vi "read_db_for_batch_processor.vi"(7 "Update Error files?":bool, 8 "error in (no error)":errorcluster, 9 "Lower Timestamp":timestamp, 10 "Upper Timestamp":timestamp, 11 "Update old files?":bool) -> (0 "error out":errorcluster, 3 "BP Array":T1[](array[typedef]) {"File Location" items=["Currently Writing"=-3, "Labview Files"=-2, "Mars Data Processing Factility"=-1, "Local Cache "=0, "Old Storage"=1, "Storage"=2]})   [LabVIEW 2012]
uses:
  Batch Processor/bp_cluster.ctl
  File_location.ctl
  <vilib>/addons/database/Auxilliary.llb/DB Tools Cursor Type.ctl
  <vilib>/addons/database/Connection.llb/Conn Execute.vi
  <vilib>/addons/database/Recordset.llb/Rec Fetch Recordset Data (R).vi
  <vilib>/addons/database/Recordset.llb/Rec Destroy - Connection.vi
  <vilib>/addons/database/_DB Variant To Data/Database Variant To Data.xnode
  <vilib>/addons/database/NI_Database_API.lvlib
panel:
  out "size(s)":i32
  out "SQL Query Sintax":string
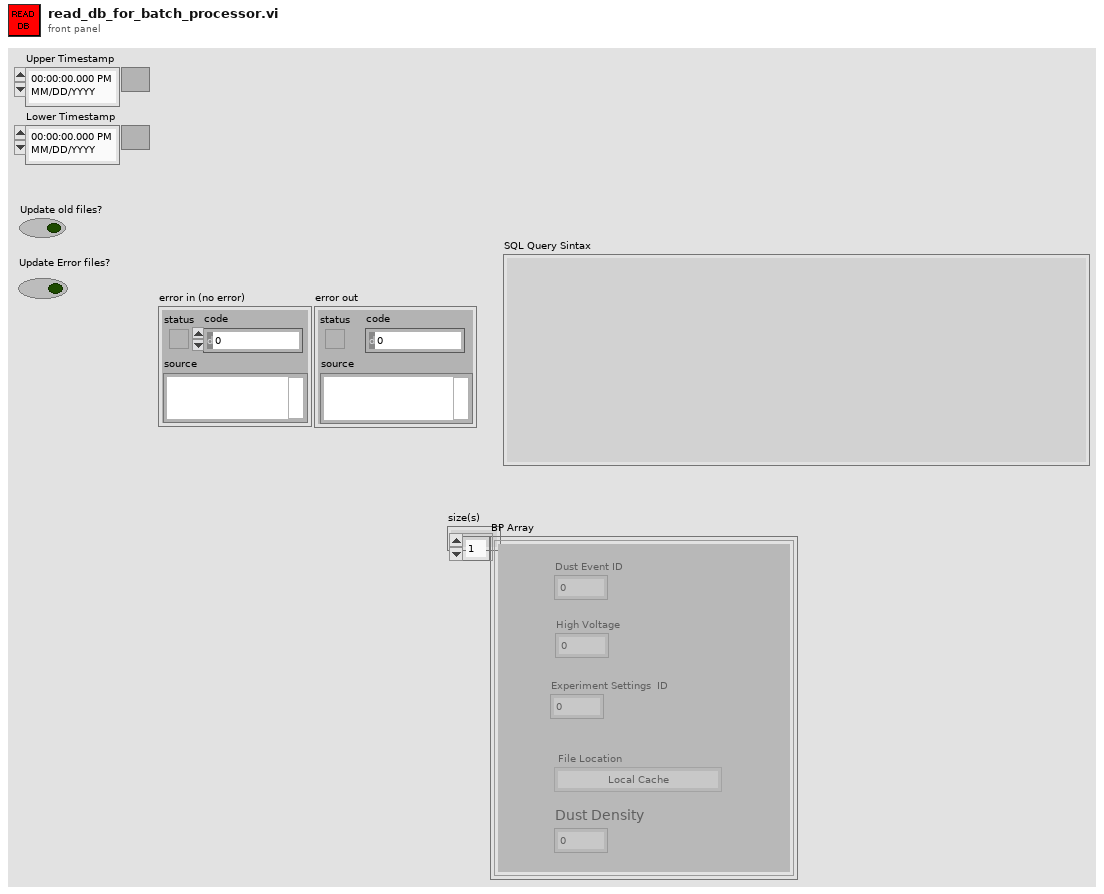
[diagram p1: front panel]
types:
  T1 = typedef "bp_cluster.ctl" = cluster{"Dust Event ID":i64, "High Voltage":sgl, "Experiment Settings  ID":i64, "File Location":T2, "Dust Density":dbl}
  T2 = typedef "File_location.ctl" = i8
  T3 = typedef "NI_Database_API.lvlib/DB Tools Cursor Type.ctl" = enum16{"forward-only", "keyset", "dynamic", "static"}
  T4 = typedef "NI_Database_API.lvlib/Conn ObjectReference.ctl" = refnum<k1>
  T5 = typedef "NI_Database_API.lvlib/Rec ObjectReference.ctl" = refnum<k1>
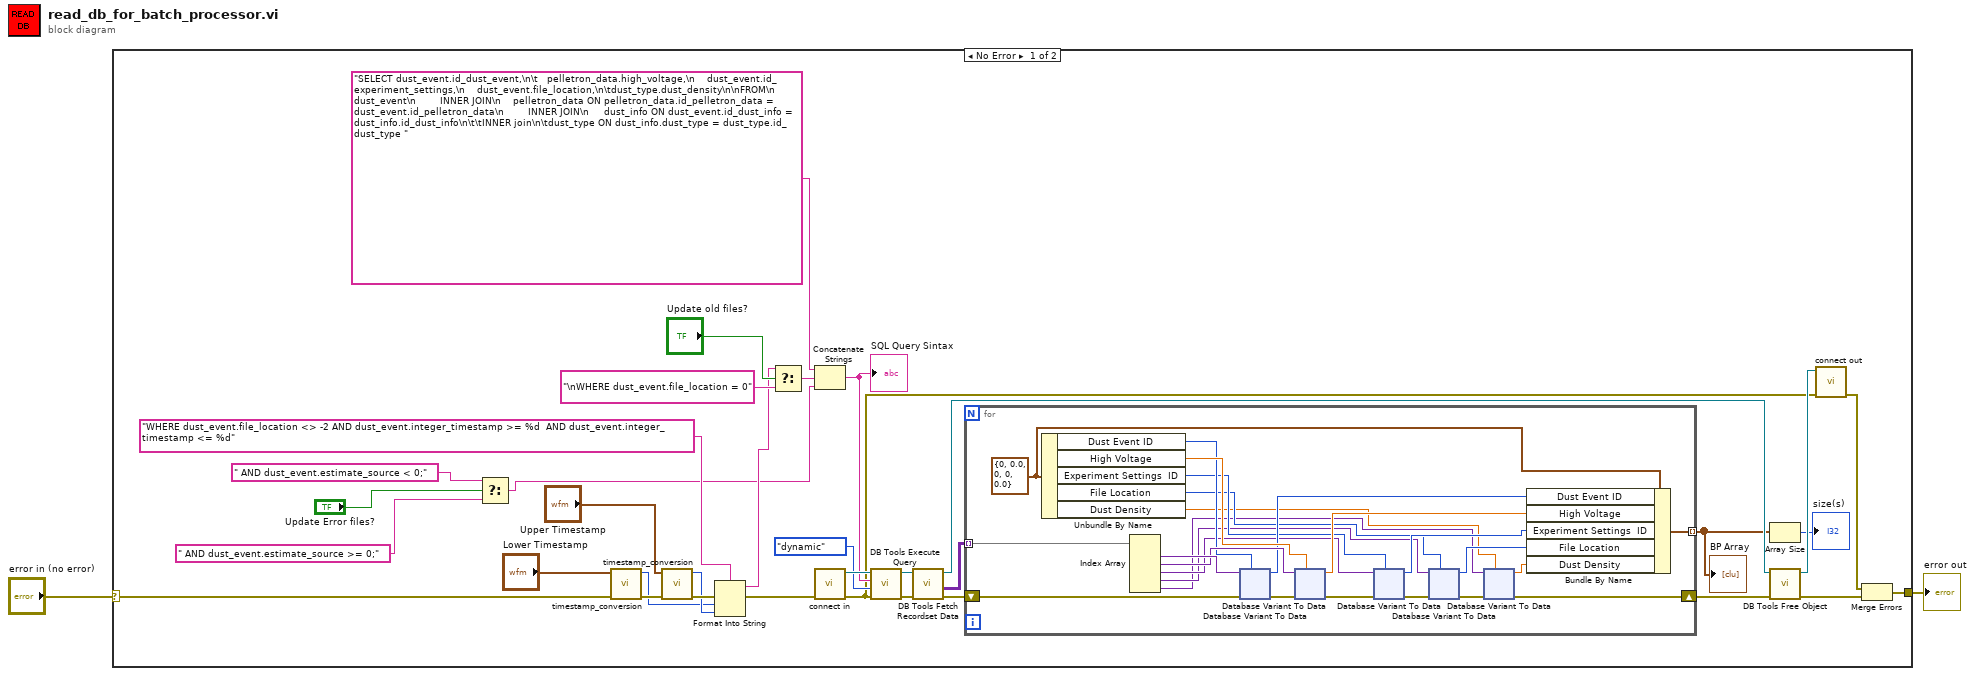
[diagram p0: block diagram]
diagram:
  n1 = case shown="No Error" "error in (no error)" {
    selector: "error in (no error)" -> [w17 w221]
    tunnel: [w11 w221] -> w1
    frame No Error {
      n2 = Select(t=" AND dust_event.estimate_source < 0;", s="Update Error files?", f=" AND dust_event.estimate_source >= 0;") -> (s? t:f=w3:string)
      n3 = call "timestamp_conversion.vi"("error in (no error)"=w17, "Time Stamp"="Lower Timestamp") -> ("error out"=w18:errorcluster, "Integer Time"=w14:i64)  [unwired: 7 in]
      n4 = call "timestamp_conversion.vi"("error in (no error)"=w18, "Time Stamp"="Upper Timestamp") -> ("error out"=w16:errorcluster, "Integer Time"=w15:i64)  [unwired: 7 in]
      n5 = Format Into String(format string="WHERE dust_event.file_location <> -2 AND dust_event.integer_timestamp >= %d  AND dust_event.integer_timestamp <= %d" ("string"), error in=w16, w14, w15) -> (resulting string=w4:string, error out=w19:errorcluster)  [unwired: 1 in]
      n6 = Select(t=w4, s="Update old files?", f="\nWHERE dust_event.file_location = 0" ("string")) -> (s? t:f=w23:string)
      n7 = Concatenate Strings("SELECT dust_event.id_dust_event,\n\t   pelletron_data.high_voltage,\n    dust_event.id_experiment_settings,\n    dust_event.file_location,\n\tdust_type.dust_density\n\nFROM\n    dust_event\n        INNER JOIN\n    pelletron_data ON pelletron_data.id_pelletron_data = dust_event.id_pelletron_data\n        INNER JOIN\n     dust_info ON dust_event.id_dust_info = dust_info.id_dust_info\n\t\tINNER join\n\tdust_type ON dust_info.dust_type = dust_type.id_dust_type " ("string"), w23, w3) -> (w25:string)
      "SQL Query Sintax" <- w25
      n8 = call "connect in.vi"("error in (no error)"=w19) -> ("error out"=w8:errorcluster, "Database Connection"=w31:T4)  [unwired: 6 in, 1 out]
      n9 = call-poly <vilib>:"DB Tools Execute Query.vi"("error in (no error)"=w8, "cursor type"=DB_Tools_Cursor_Type."dynamic", "SQL query"=w25, "connection reference"=w31) -> ("error out"=w35:errorcluster, "recordset reference"=w36:T5)  [unwired: 4 in]
      n10 = call-poly <vilib>:"DB Tools Fetch Recordset Data.vi"("error in (no error)"=w35, "recordset reference"=w36) -> ("error out"=w33:errorcluster, "recordset data"=w29:variant[][], "recordset reference out"=w34:T5)  [unwired: 3 in]
      n11 = for {
        tunnel: w29 -> [w60] mode=indexing
        shift-right: [w37] -> w32
        shift-left: w33 -> [w59]
        tunnel: [w55] -> w27 mode=indexing
        w50 = T1 {"Dust Event ID"=0, "High Voltage"=0.0, "Experiment Settings  ID"=0, "File Location"=0, "Dust Density"=0.0} ("Batch Processing Cluster")
        n12 = Unbundle By Name(w50) -> ("Dust Event ID"=w52:i64, "High Voltage"=w53:sgl, "Experiment Settings  ID"=w48:i64, "File Location"=w43:T2, "Dust Density"=w40:dbl)
        n13 = Index Array(array=w60) -> (element #1=w58:variant, element #2=w57:variant, element #3=w49:variant, element #4=w45:variant, element #5=w39:variant)  [unwired: 5 in]
        n14 = xnode "Database Variant To Data"("database variant"=w58, "error in"=w59, "type"=w52) -> ("data"=w51:i64, "error out"=w56:errorcluster)
        n15 = xnode "Database Variant To Data"("database variant"=w57, "error in"=w56, "type"=w53) -> ("data"=w54:sgl, "error out"=w46:errorcluster)
        n16 = xnode "Database Variant To Data"("database variant"=w49, "error in"=w46, "type"=w48) -> ("data"=w47:i64, "error out"=w44:errorcluster)
        n17 = xnode "Database Variant To Data"("database variant"=w45, "error in (no error)"=w44, "type"=w43) -> ("data"=w42:T2, "error out"=w41:errorcluster)
        n18 = xnode "Database Variant To Data"("database variant"=w39, "error in"=w41, "type"=w40) -> ("data"=w38:dbl, "error out"=w37:errorcluster)
        n19 = Bundle By Name(cluster=w50, "Dust Event ID"=w51, "High Voltage"=w54, "Experiment Settings  ID"=w47, "File Location"=w42, "Dust Density"=w38) -> (w55:T1)
      }
      "BP Array" <- w27
      n20 = Array Size(array=w27) -> (size(s)=→"size(s)":i32)
      n21 = call-poly <vilib>:"DB Tools Free Object.vi"("error in (no error)"=w32, "recordset reference"=w34) -> ("error out"=w9:errorcluster, "connection reference"=w30:T4)  [unwired: 8 in]
      n22 = call "connect out.vi"("error in (no error)"=w8, "connection reference"=w30) -> ("error out"=w10:errorcluster)  [unwired: 9 in]
      n23 = Merge Errors(w10, w9) -> (w11:errorcluster)
    }
    frame Error {
    }
  }
  "error out" <- w1
